vi "SA WIN Cloud Toolkit Main.vi"() -> ()   [LabVIEW 2017]
doc: "Example AWS toolkit API calls to learn more about how they work. \n\nJames Tillett PE\nEndeavor Engineering Inc.\nwww.endeavoreng.com"
uses:
  <vilib>/AWS Toolkit/Core/HTTP Request/Region.ctl
  <vilib>/AWS Toolkit/Core/HTTP Request/AWS Credentials.ctl
  <vilib>/AWS Toolkit/SNS/Phone Number/Phone Number.lvclass
  <vilib>/AWS Toolkit/S3/Bucket/Bucket.lvclass
  <vilib>/AWS Toolkit/SQS/Queue/Queue.lvclass
  <vilib>/AWS Toolkit/Core/HTTP Request/HTTP Request.lvclass
panel:
  in  "Delete SQS Msg After Receipt":bool
  out "SNS Messages":string
  in  "Enable SNS Msg to SQS":bool
  out "MD5 of Body":string="fffb3eb6649c80efe5a027f4c4a5ef23"
  out "Message ID":string="4a0cf352-e98d-437e-9363-23ecd7bf3de7"
  in  "Message Body":string="One step for me - giant leap for Endeavor."
  in  "Queue Name":string="mynicloud-demotest2"
  in  "Send to SQS":bool
  out "ETag":string="059d033624a7a76be0d5e37e09eab1dd-1"
  out "Location":string="https://mynicloud-demo.s3-us-west-2.amazonaws.com/niweekdemo/JournalClientError.txt"
  in  "Object Bucket":string="mynicloud-demotest2"
  in  "Object Path":string="niiotdemo/AWSToolkitTestFile.txt"
  in  "File to Upload":path=path "E:/Bitbucket/sbrio-eval-ni-iot-examples/sbRIO Eval Example Code/sbRIO Eval IoT Example Code/AWSTookitTestFile.txt"
  in  "Send File to S3":bool
  in  "stop":bool
  in  "Message Out":string
  in  "AWS Credentials":T1={"Access Key"="AKIAJHAPAD6QJ2EDKQBA", "Secret Key"="AHlHUPw/PucMyDtRCgPh4o+m/Eu1u91KOthIJkOX"}
  in  "Region":T2=enum."us-west-2"
  in  "Phone Number":string="+15037066913"
  in  "Send SMS Direct":bool
  # "SNS"
  # "S3"
  # "SQS"
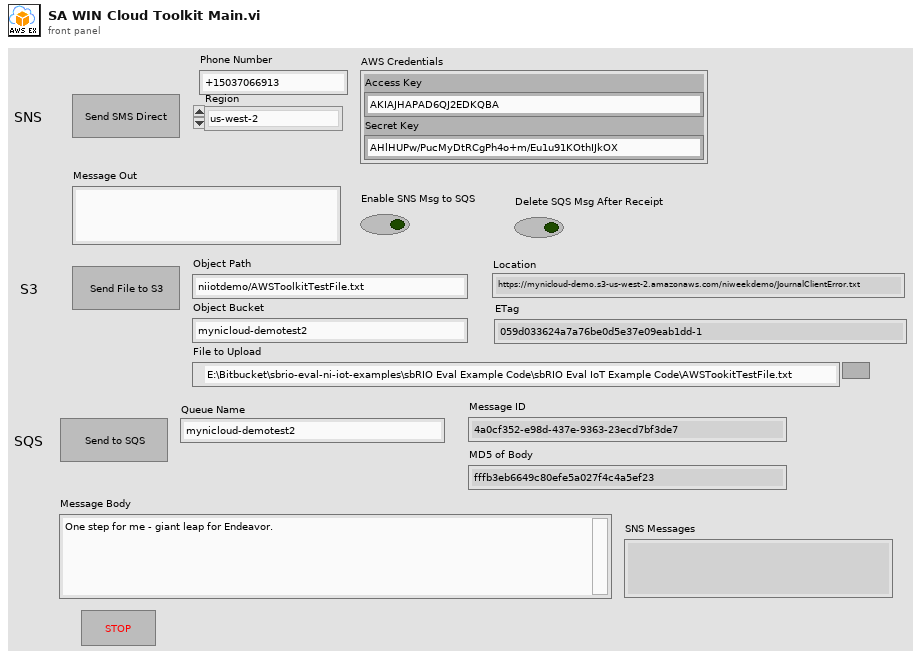
[diagram p1: front panel]
types:
  T1 = typedef "NI_AWS_Core.lvlib/HTTP Request.lvclass/AWS Credentials.ctl" = cluster{"Access Key":string, "Secret Key":string}
  T2 = typedef "NI_AWS_Core.lvlib/HTTP Request.lvclass/Region.ctl" = enum16{"us-east-1", "us-east-2", "us-west-1", "us-west-2", "ap-northeast-1", "ap-northeast-2", "ap-southeast-1", "ap-southeast-2", "ca-central-1", "eu-central-1", "eu-west-1", "eu-west-2", "sa-east-1"}
  T3 = typedef "NI_AWS_SQS.lvlib/Queue.lvclass/Message.ctl" = cluster{"Body":string, "MD5 of Body":string, "ID":string, "Receipt Handle":string, "Native Attributes":T4[], "Custom Attributes":T6[], "MD5 of Custom Attributes":string}
  T4 = typedef "NI_AWS_SQS.lvlib/Queue.lvclass/Message Attribute Value Pair.ctl" = cluster{"Attribute":T5, "Value":string}
  T5 = typedef "NI_AWS_SQS.lvlib/Queue.lvclass/Message Attribute.ctl" = enum16{"SenderId", "SentTimestamp", "ApproximateReceiveCount", "ApproximateFirstReceiveTimestamp"}
  T6 = typedef "NI_AWS_SQS.lvlib/Queue.lvclass/Custom Attribute.ctl" = cluster{"Name":string, "Type":T7, "Value":string}
  T7 = typedef "NI_AWS_SQS.lvlib/Queue.lvclass/Custom Attribute Type.ctl" = enum16{"String", "Number", "Binary"}
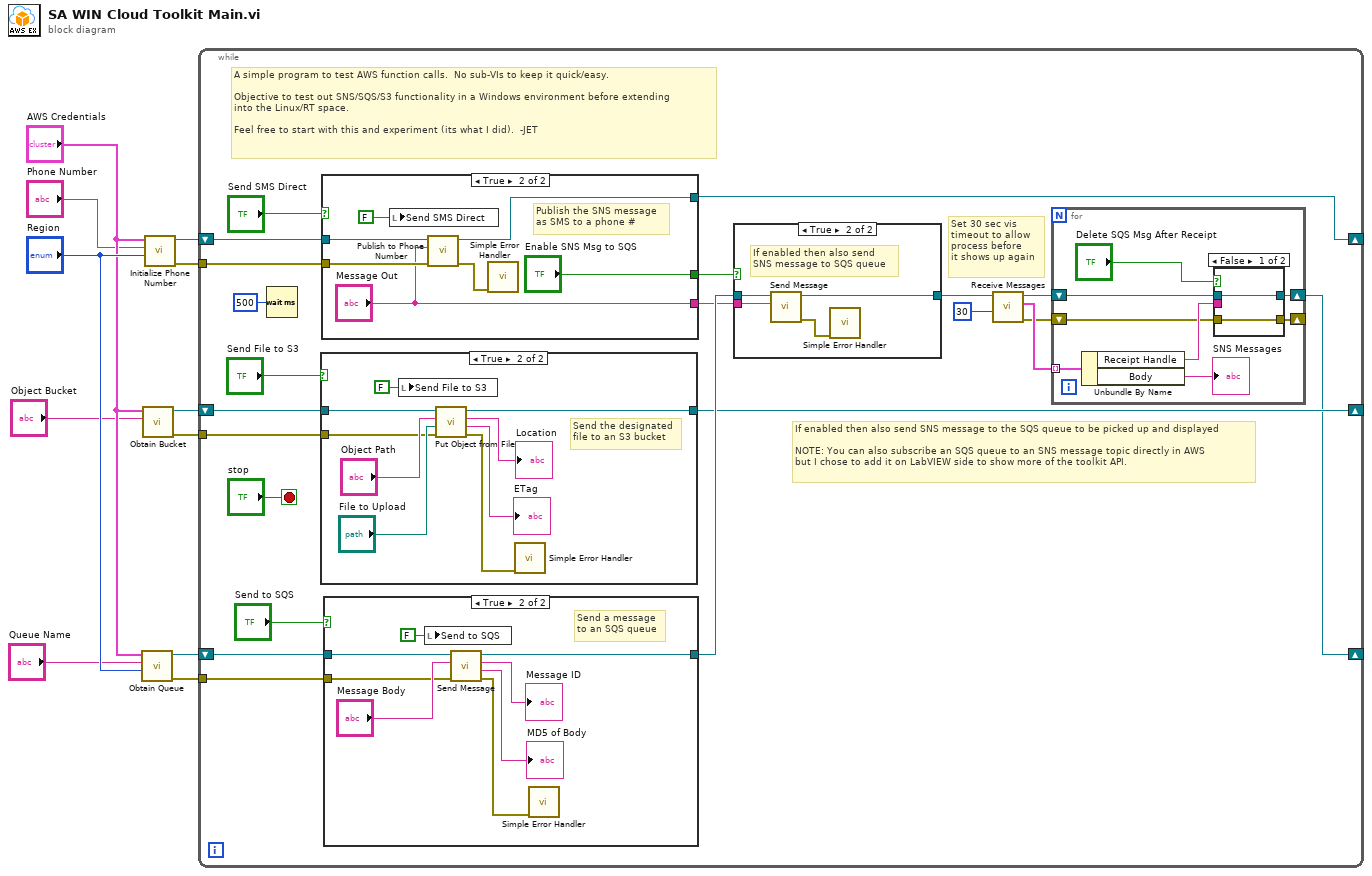
[diagram p0: block diagram]
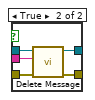
[diagram p2: hidden frame]
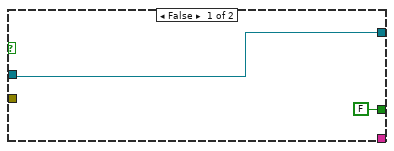
[diagram p6: hidden frame]
diagram:
  n1 = call <vilib>:"Obtain Queue.vi"("Region"="Region", "Name"="Queue Name", "AWS Credentials"="AWS Credentials") -> ("error out"=w6:errorcluster, "SQS"=w5:refnum<class "Queue.lvclass">)  [unwired: 7 in]
  n2 = call <vilib>:"Obtain Bucket.vi"("Bucket name"="Object Bucket", "AWS Credentials"="AWS Credentials") -> ("error out"=w4:errorcluster, "Bucket"=w3:refnum<class "Bucket.lvclass">)  [unwired: 8 in]
  n3 = call <vilib>:"Initialize Phone Number.vi"("Region"="Region", "Phone Number"="Phone Number", "AWS Credentials"="AWS Credentials") -> ("error out"=w2:errorcluster, "Phone Number"=w1:refnum<class "Phone Number.lvclass">)  [unwired: 7 in]
  n4 = while {
    tunnel: w6 -> [w26]
    tunnel: w4 -> [w24]
    tunnel: w2 -> [w22]
    shift-right: [w15] -> _
    shift-left: w1 -> [w21]
    shift-right: [w14] -> _
    shift-left: w3 -> [w23]
    shift-right: [w13] -> _
    shift-left: w5 -> [w25]
    stop <- "stop" stop-if-true
    # "Set 30 sec vis\ntimeout to allow\nprocess before\nit shows up again"
    # "If enabled then also send SNS message to the SQS queue to be picked up and displayed\n\nNOTE: You can also subscribe an SQS queue to an SNS message topic directly in AWS\nbut I chose to add it on LabVIEW side to show more of the toolkit API."
    # "A simple program to test AWS function calls.  No sub-VIs to keep it quick/easy.\n\nObjective to test out SNS/SQS/S3 functionality in a Windows environment before extending\ninto the Linux/RT space.  \n\nFeel free to start with this and experiment (its what I did).  -JET"
    n5 = Wait (ms)(milliseconds to wait=u32 500) -> ()  [unwired: 1 out]
    n6 = case shown="True" "Send File to S3" {
      tunnel: w24 -> [_ w66]
      tunnel: w23 -> [w63 w65]
      tunnel: [w63 w64] -> w14
      frame False {
      }
      frame True {
        # "Send the designated\nfile to an S3 bucket"
        n7 = local write "Send File to S3"(FALSE ("Send File to S3")) -> ()
        n8 = call <vilib>:"Put Object from File.vi"("error in (no error)"=w66, "File"="File to Upload", "Object Path"="Object Path", "Bucket in"=w65) -> ("error out"=w67:errorcluster, "ETag"=→"ETag":string, "Location"=→"Location":string, "Bucket out"=w64:refnum<class "Bucket.lvclass">)  [unwired: 3 in, 1 out]
        n9 = call <vilib>:"Simple Error Handler.vi"("error in (no error)"=w67) -> ()  [unwired: 4 in, 5 out]
      }
    }
    n10 = case shown="True" "Send SMS Direct" {
      tunnel: w22 -> [_ w79]
      tunnel: w21 -> [w73 w78]
      tunnel: [FALSE ("Enable SNS Msg to SQS") "Enable SNS Msg to SQS"] -> w29
      tunnel: [_ "Message Out"] -> w27
      tunnel: [w73 w75] -> w15
      frame False {
      }
      frame True {
        # "Publish the SNS message\nas SMS to a phone #"
        n11 = local write "Send SMS Direct"(FALSE ("Send SMS")) -> ()
        n12 = call <vilib>:"Publish to Phone Number.vi"("error in (no error)"=w79, "Message"="Message Out", "Phone Number in"=w78) -> ("error out"=w80:errorcluster, "Phone Number out"=w75:refnum<class "Phone Number.lvclass">)  [unwired: 7 in]
        n13 = call <vilib>:"Simple Error Handler.vi"("error in (no error)"=w80) -> ()  [unwired: 4 in, 5 out]
      }
    }
    n14 = case shown="True" "Send to SQS" {
      tunnel: w26 -> [_ w57]
      tunnel: w25 -> [w54 w56]
      tunnel: [w54 w55] -> w28
      frame False {
      }
      frame True {
        # "Send a message\nto an SQS queue"
        n15 = local write "Send to SQS"(FALSE ("Send to SQS")) -> ()
        n16 = call <vilib>:"Send Message.vi"("error in (no error)"=w57, "Message Body"="Message Body", "SQS in"=w56) -> ("error out"=w61:errorcluster, "MD5 of Body"=→"MD5 of Body":string, "Message ID"=→"Message ID":string, "SQS out"=w55:refnum<class "Queue.lvclass">)  [unwired: 4 in, 1 out]
        n17 = call <vilib>:"Simple Error Handler.vi"("error in (no error)"=w61) -> ()  [unwired: 4 in, 5 out]
      }
    }
    n18 = case shown="True" w29 {
      tunnel: w28 -> [w49 w53]
      tunnel: w27 -> [_ w52]
      tunnel: [w49 w50] -> w20
      frame False {
      }
      frame True {
        # "If enabled then also send\nSNS message to SQS queue"
        n19 = call <vilib>:"Send Message.vi"("Message Body"=w52, "SQS in"=w53) -> ("error out"=w51:errorcluster, "SQS out"=w50:refnum<class "Queue.lvclass">)  [unwired: 5 in, 3 out]
        n20 = call <vilib>:"Simple Error Handler.vi"("error in (no error)"=w51) -> ()  [unwired: 4 in, 5 out]
      }
    }
    n21 = call <vilib>:"Receive Messages.vi"("Visibility Timeout"=30, "SQS in"=w20) -> ("error out"=w16:errorcluster, "Messages"=w18:T3[], "SQS out"=w17:refnum<class "Queue.lvclass">)  [unwired: 7 in]
    n22 = for {
      tunnel: w18 -> [w41] mode=indexing
      shift-right: [w36] -> w13
      shift-left: w17 -> [w39]
      shift-right: [w35] -> _
      shift-left: w16 -> [w37]
      n23 = Unbundle By Name(w41) -> ("Receipt Handle"=w38:string, "Body"=→"SNS Messages":string)
      n24 = case shown="False" "Delete SQS Msg After Receipt" {
        tunnel: w39 -> [w43 w48]
        tunnel: w38 -> [_ w47]
        tunnel: w37 -> [w42 w46]
        tunnel: [w43 w45] -> w36
        tunnel: [w42 w44] -> w35
        frame False {
        }
        frame True {
          n25 = call <vilib>:"Delete Message.vi"("error in (no error)"=w46, "Receipt Handle"=w47, "SQS in"=w48) -> ("error out"=w44:errorcluster, "SQS out"=w45:refnum<class "Queue.lvclass">)  [unwired: 7 in]
        }
      }
    }
  }
